vi "makeInitializeDD.vi"(0 "vi refnum":refnum<vi>, 1 "Visitor class path":path, 2 "error in":errorcluster) -> (3 "vi refnum":refnum<vi>, 6 "error out":errorcluster)   [LabVIEW 2009, in "HGF_VisitorGenerator.lvlib"]
doc: "replace visitor class controls of init.vi and make VI dynamic dispatch"
uses:
  HGF_VisitorGenerator.lvlib
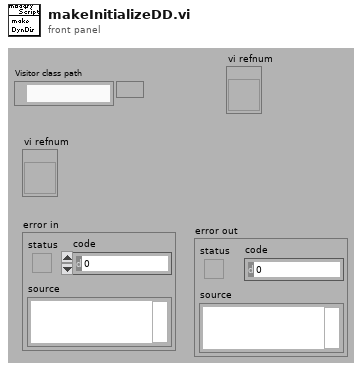
[diagram p1: front panel]
types:
  T1 = enum16{"Invalid Wire Rule", "Required", "Recommended", "Optional", "Dynamic Dispatch"}
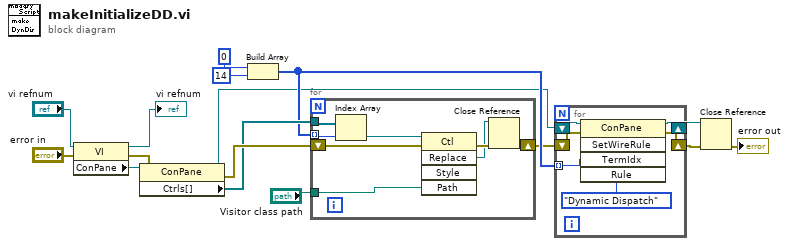
[diagram p0: block diagram]
diagram:
  n1 = property class="VI"(reference="vi refnum", error in="error in") -> (reference out=→"vi refnum":refnum<vi>, error out=w16:errorcluster, "ConPane"=w12:refnum<vi>)
  n2 = property class="ConPane"(reference=w12, error in=w16) -> (reference out=w4:refnum<vi>, error out=w9:errorcluster, "Ctrls[]"=w6:refnum<vi>[])
  n3 = Build Array(0 ("index"), 14 ("index")) -> (w5:i32[])
  n4 = for {
    tunnel: "Visitor class path" -> [w24]
    shift-right: [w23] -> w2
    shift-left: w9 -> [w20]
    tunnel: w6 -> [w19]
    tunnel: w5 -> [w17] mode=indexing
    n5 = Index Array(array=w19, index=w17) -> (element=w18:refnum<vi>)
    n6 = invoke class="Ctl" method="Replace"(reference=w18, error in=w20, "Path"=w24) -> (error out=w22:errorcluster, "Replace"=w21:refnum<vi>)  [unwired: 2 in, 3 out]
    n7 = Close Reference(reference=w21, error in (no error)=w22) -> (error out=w23:errorcluster)
  }
  n8 = for {
    shift-right: [w29] -> w3
    shift-left: w4 -> [w30]
    tunnel: w5 -> [w26] mode=indexing
    shift-right: [w25] -> w1
    shift-left: w2 -> [w28]
    n9 = invoke class="ConPane" method="SetWireRule"(reference=w30, error in=w28, "TermIdx"=w26, "Rule"=T1."Dynamic Dispatch" ("new element/subarray")) -> (reference out=w29:refnum<vi>, error out=w25:errorcluster)  [unwired: 1 in, 3 out]
  }
  n10 = Close Reference(reference=w3, error in (no error)=w1) -> (error out=→"error out":errorcluster)
